vi "DetermineChangeToTiming.vi"(10 "OldVal":T2 {"Timing Sequence"."Dt" format="%_3p"; "Timing Sequence"."Time" format="%_3p"}, 11 "NewVal":T2 {"Timing Sequence"."Dt" format="%_3p"; "Timing Sequence"."Time" format="%_3p"}) -> (2 "Position":cluster{"Card":dbl, "Channel":dbl}, 3 "Job":T1(ring))   [LabVIEW 2013]
doc: "Determines the change to the timing cluster that generated the event and prepares a job.\n\nThe change in the timing cluster is determined by comparing old and new values of each elment fo the timing cluster. It is assumed that only one value can change per event. i.e. the computer can process events faster than the user can generate them. \nThe VI prepares a job for the consumer loop to do with information on where the change occured."
uses:
  Controls/TimingControlArray.ctl
  Controls/TimingControl.ctl
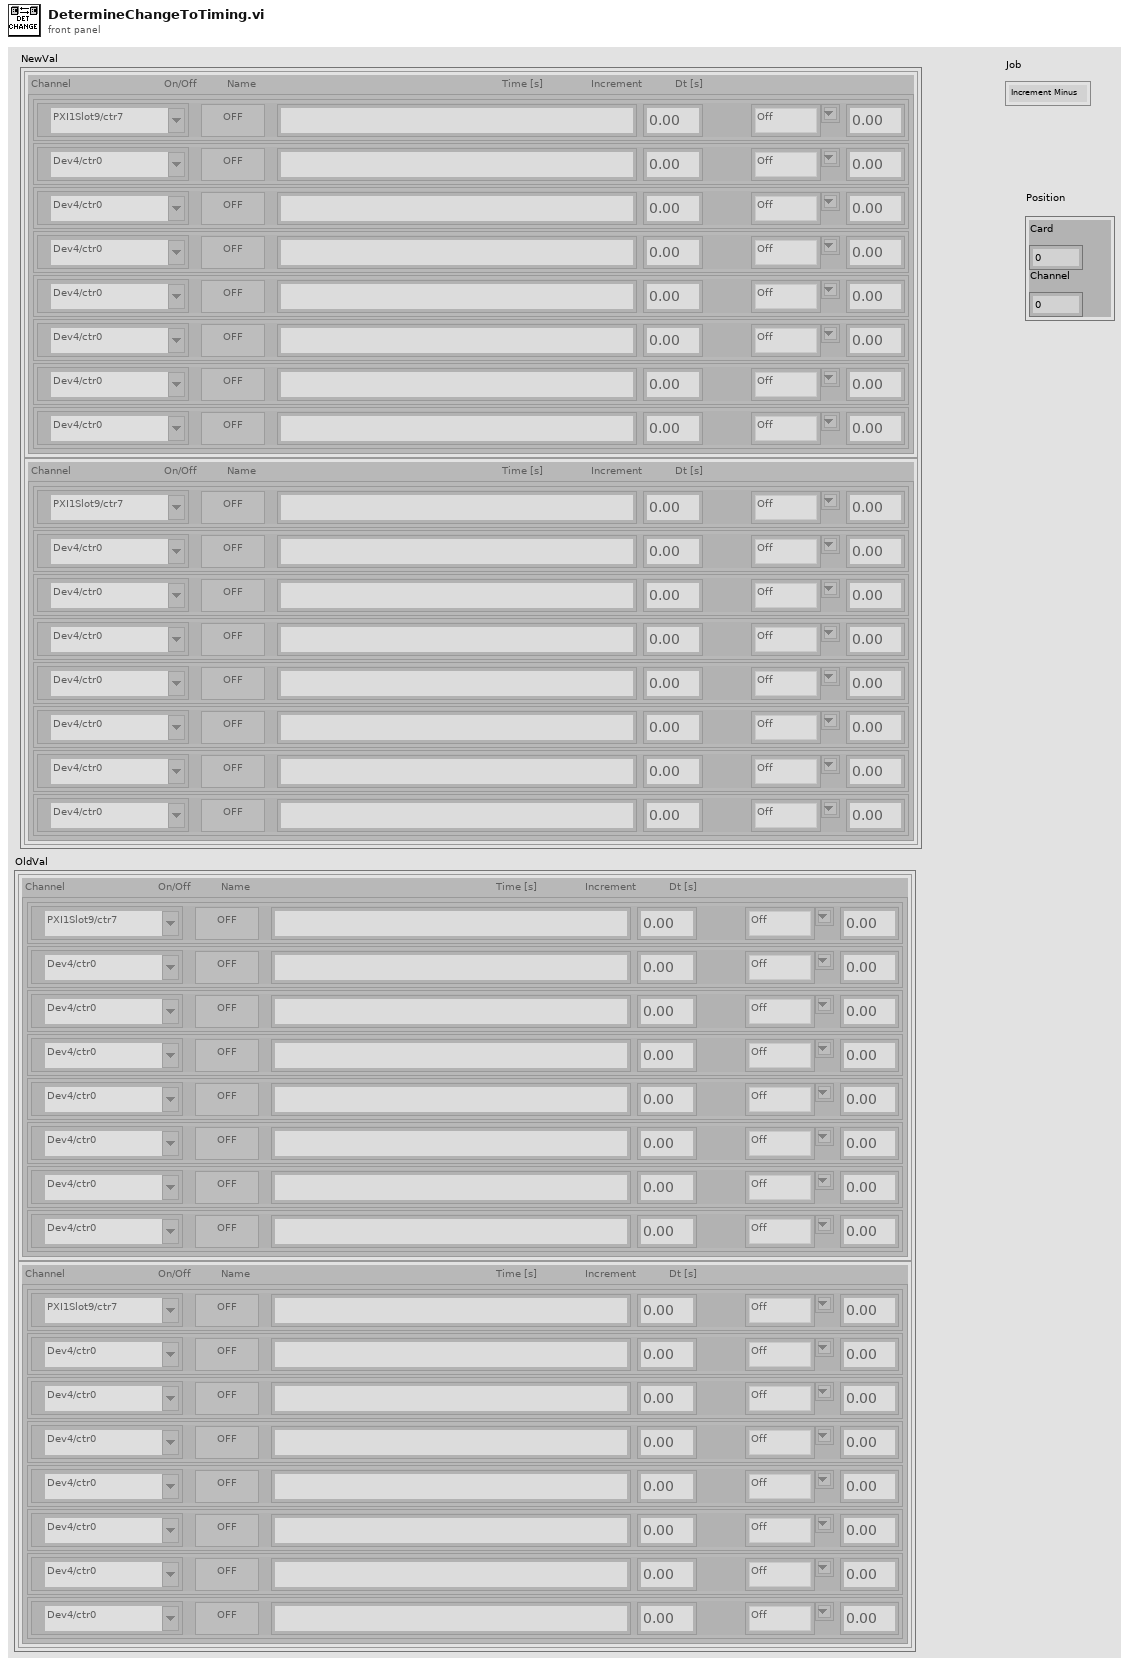
[diagram p1: front panel]
types:
  T1 = enum16{"Increment Minus", "Increment Add", "Enable/Dis", "Redraw Timing Plot", "Do Nothing"}
  T2 = typedef "TimingControlArray.ctl" = T3[]
  T3 = typedef "TimingControl.ctl" = cluster{"Timing Sequence":cluster{"Active":bool, "counter":tag, "Channel Name":string, "Time":dbl, "Increment":string, "Dt":dbl}[]}
  T4 = cluster{"Timing Sequence":cluster{"Active":bool, "counter":bool, "Channel Name":bool, "Time":bool, "Increment":bool, "Dt":bool}[]}[]
  T5 = cluster{"Active":bool, "counter":bool, "Channel Name":bool, "Time":bool, "Increment":bool, "Dt":bool}[]
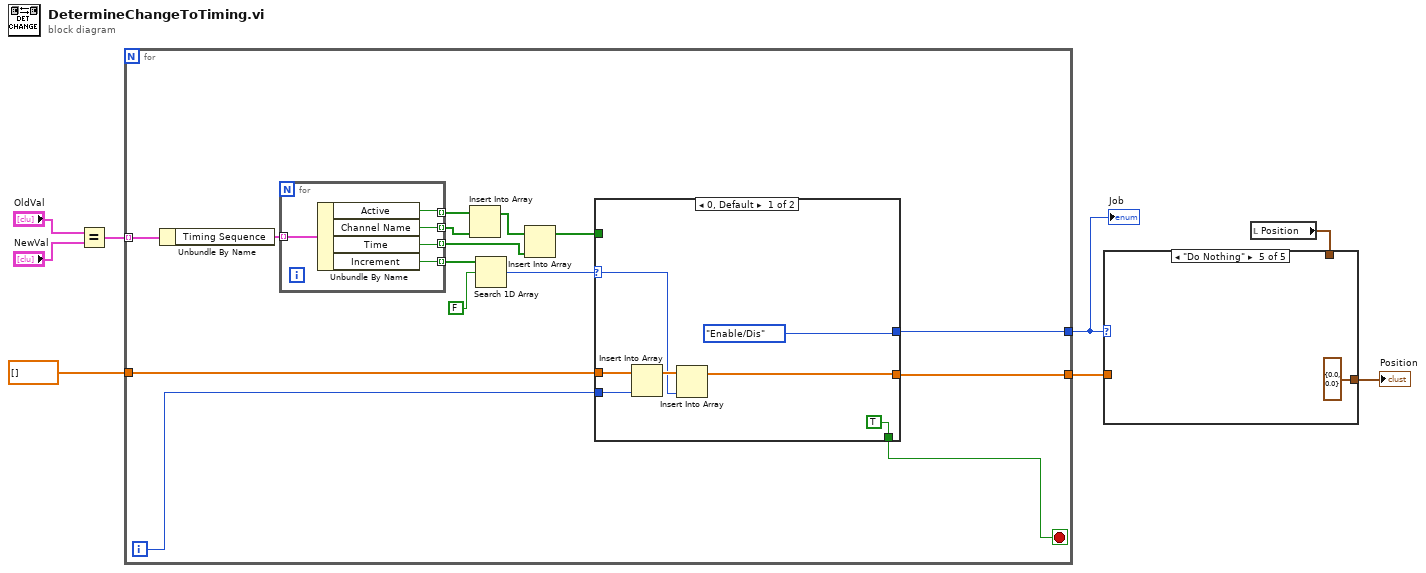
[diagram p0: block diagram]
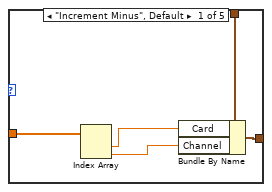
[diagram p2: hidden frame]
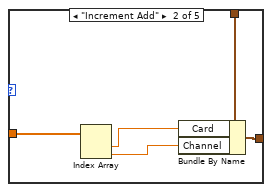
[diagram p3: hidden frame]
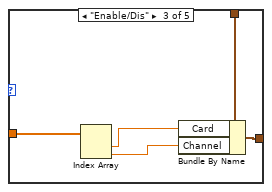
[diagram p4: hidden frame]
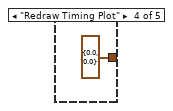
[diagram p5: hidden frame]
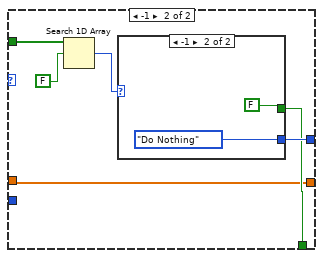
[diagram p6: hidden frame]
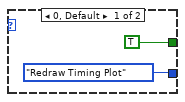
[diagram p7: hidden frame]
diagram:
  n1 = Equal?(x="OldVal", y="NewVal") -> (x = y?=w6:T4)
  n2 = for {
    tunnel: w6 -> [w9] mode=indexing
    tunnel: [w23] -> w4
    tunnel: [w22] -> w3
    tunnel: dbl[] [] ("Location") -> [w21]
    i -> [w20]
    stop <- w19 stop-if-true
    n3 = Unbundle By Name(w9) -> ("Timing Sequence"=w18:T5)
    n4 = for {
      tunnel: w18 -> [w45] mode=indexing
      tunnel: [w44] -> w14 mode=indexing
      tunnel: [w43] -> w13 mode=indexing
      tunnel: [w42] -> w11 mode=indexing
      tunnel: [w41] -> w17 mode=indexing
      n5 = Unbundle By Name(w45) -> ("Active"=w44:bool, "Channel Name"=w43:bool, "Time"=w42:bool, "Increment"=w41:bool)
    }
    n6 = Insert Into Array(array=w14, new element=w13) -> (w12:bool[])  [unwired: 1 in]
    n7 = Search 1D Array(1D array=w17, element=FALSE) -> (index of element=w15:i32)  [unwired: 1 in]
    n8 = Insert Into Array(array=w12, new element=w11) -> (w10:bool[])  [unwired: 1 in]
    n9 = case shown="0, Default" w15 {
      selector: w15 -> [w25 _]
      tunnel: w10 -> [_ w36]
      tunnel: [T1."Enable/Dis" w33] -> w23
      tunnel: [w24 w31] -> w22
      tunnel: w21 -> [w28 w31]
      tunnel: w20 -> [w27 _]
      tunnel: [TRUE w32] -> w19
      frame 0, Default {
        n10 = Insert Into Array(array=w28, new element=w27) -> (w26:dbl[])  [unwired: 1 in]
        n11 = Insert Into Array(array=w26, new element=w25) -> (w24:dbl[])  [unwired: 1 in]
      }
      frame -1 {
        n12 = Search 1D Array(1D array=w36, element=FALSE) -> (index of element=w34:i32)  [unwired: 1 in]
        n13 = case shown="-1" w34 {
          tunnel: [T1."Redraw Timing Plot" T1."Do Nothing"] -> w33
          tunnel: [TRUE FALSE] -> w32
          frame 0, Default {
          }
          frame -1 {
          }
        }
      }
    }
  }
  "Job" <- w4
  n14 = local read "Position"() -> (w2:cluster{"Card":dbl, "Channel":dbl})
  n15 = case shown="\"Do Nothing\"" w4 {
    tunnel: w3 -> [w50 w55 w60 _ _]
    tunnel: w2 -> [w49 w54 w59 _ _]
    tunnel: [w46 w51 w56 cluster{"Card":dbl, "Channel":dbl} {"Card"=0.0, "Channel"=0.0} ("Position") cluster{"Card":dbl, "Channel":dbl} {"Card"=0.0, "Channel"=0.0} ("Position")] -> w1
    frame "Increment Minus", Default {
      n16 = Index Array(array=w50) -> (element #1=w48:dbl, element #2=w47:dbl)  [unwired: 2 in]
      n17 = Bundle By Name(cluster=w49, "Card"=w48, "Channel"=w47) -> (w46:cluster{"Card":dbl, "Channel":dbl})
    }
    frame "Increment Add" {
      n18 = Index Array(array=w55) -> (element #1=w53:dbl, element #2=w52:dbl)  [unwired: 2 in]
      n19 = Bundle By Name(cluster=w54, "Card"=w53, "Channel"=w52) -> (w51:cluster{"Card":dbl, "Channel":dbl})
    }
    frame "Enable/Dis" {
      n20 = Index Array(array=w60) -> (element #1=w58:dbl, element #2=w57:dbl)  [unwired: 2 in]
      n21 = Bundle By Name(cluster=w59, "Card"=w58, "Channel"=w57) -> (w56:cluster{"Card":dbl, "Channel":dbl})
    }
    frame "Redraw Timing Plot" {
    }
    frame "Do Nothing" {
    }
  }
  "Position" <- w1
